vi "get_value.vi"() -> ()   [LabVIEW 2019]
uses:
  Global.vi
panel:
  in  "stop":bool
  out "spill_id_global":i64
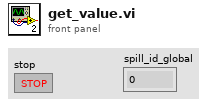
[diagram p1: front panel]
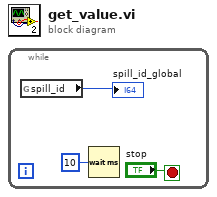
[diagram p0: block diagram]
diagram:
  n1 = while {
    stop <- "stop" stop-if-true
    n2 = global read "Global.vi" "spill_id"() -> (→"spill_id_global":i64)
    n3 = Wait (ms)(milliseconds to wait=u32 10) -> ()  [unwired: 1 out]
  }
